vi "Add Caption and Table.vi"(0 "PDF Report IN":T21(xcontrol), 5 "Caption":string, 7 "PdfPTable":refnum<k24>, 11 "error in (no error)":errorcluster) -> (4 "PDF Report OUT":T21(xcontrol), 14 "ms":u32, 15 "error out":errorcluster)   [LabVIEW 2012]
doc: "Version 1.0\nDeveloped by Jean-Marc Simard\nCopyright © 2010, Exaprom Inc.\nAll rights reserved.\nLicense: BSD\n\nWith iTextSharp 4.1.6 (http://itextsharp.sourceforge.net)\nunder Mozilla Public License Version 1.1\n(http://www.mozilla.org/MPL/MPL-1.1.html)"
uses:
  Controls/PDF Report Xcontrol/PDF Report.xctl
  C:/Users/MaxCorp/Documents/TopPerm - Base/DLL/itextsharp.dll
  DLL/itextsharp.dll
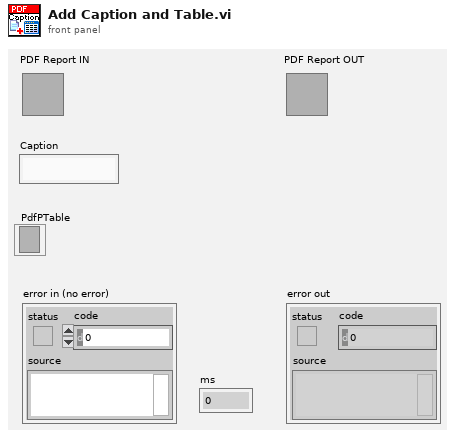
[diagram p1: front panel]
types:
  T1 = typedef "Font cluster.ctl" = cluster{"Name":string, "Size":T2, "Color":T3, "Style":cluster{"Bold":bool, "Italic":bool, "Underline":bool, "Strikeout":bool}}
  T2 = typedef "Font size.ctl" = sgl
  T3 = typedef "Font color.ctl" = u32
  T4 = typedef "Unit.ctl" = enum16{"inch", "mm"}
  T5 = typedef "Paragraphe cluster.ctl" = cluster{" Aligment":T6, "Line spacing":T7}
  T6 = typedef "Texte alignement.ctl" = enum16{"Select", "CENTER", "JUSTIFY", "LEFT", "RIGHT"}
  T7 = typedef "Line spacing.ctl" = enum16{"Select", "1.0", "1.5", "2.0"}
  T8 = typedef "Page dimensions.ctl" = cluster{"Start at page":i32, "Orientation":T9, "widht":sgl, "height":sgl, "Margin left":sgl, "Margin right":sgl, "Margin top":sgl, "Margin bottom":sgl}
  T9 = typedef "Page Orientation.ctl" = enum16{"Portrait", "Landscape"}
  T10 = typedef "Image or Table Caption.ctl" = cluster{"Caption":string, "Separator":string, "Position":enum16{"Above", "Below"}}
  T11 = typedef "Header Footer [ ].ctl" = T12[]
  T12 = typedef "Header Footer cluster.ctl" = cluster{"Start page":i32, "Type":T13, "Alignment":T14, "Vertical Alignement":T15, "Image (%)":sgl, "Page #":T16, "Text":string, "Path":string, "Font":T1, "Font refnum":refnum<k24>, "Line":cluster{"Line":T17, "Thickness (points)":sgl, "Colour":T3}}
  T13 = typedef "Header Footer Type.ctl" = enum16{"Select", "Text", "Text + hyperlink", "Page number", "Image", "Image + hyperlink"}
  T14 = typedef "Header footer horiz alignment.ctl" = enum16{"Left", "Center", "Right"}
  T15 = typedef "Cell Vertical alignment.ctl" = enum16{"TOP", "MIDDLE", "BOTTOM"}
  T16 = typedef "Page number.ctl" = cluster{"Text 1":string, "Text 2":string, "Text 3":string}
  T17 = typedef "Header Footer Line.ctl" = enum16{"No line", "Horizontal line"}
  T18 = typedef "Watermark cluster2.ctl" = cluster{"Show? (F)":bool, "Type":enum16{"Image", "Text"}, "Opacity (%)":sgl, "Rotate(°)":sgl, "Position":cluster{"Position":T19, "X":sgl, "Y":sgl}, "Image path":path, "Scaled(%)":sgl, "Image refnum":refnum<k24>, "Text":string, "Font":cluster{"Name":string, "Size":T2, "Color":T3}, "Font refnum":refnum<k24>, "Alignment":T14, "Automatic":bool}
  T19 = typedef "Watermark Position.ctl" = enum16{"Absolute", "Center (page)", "Center (text section)"}
  T20 = typedef "System Fonts.ctl" = cluster{"Font name [ ]":string[], "Font and file names [ ]":cluster{"Font name":string, "File name":string}[]}
  T21 = cluster{"Document":refnum<k24>, "Writer":refnum<k24>, "Default Font":refnum<k24>, "Default Font cluster":T1, "Path":path, "Unit (default = mm)":T4, "Paragraphe cluster":T5, "Pages dimensions [ ]":T8[], "Captions":cluster{"Image":T10, "Image counter":u16, "Table":T10, "Table counter":u16, "Font":T1}, "Header":T11, "Footer":T11, "Watermark ":T18, "Actual VI name":string, "System Fonts":T20}
  T22 = cluster{"HorizontalAlignment":i32, "SpacingBefore":sgl, "SpacingAfter":sgl}
  T23 = cluster{"HorizontalAlignment":i32, "SpacingAfter":sgl, "SpacingAfter":sgl}
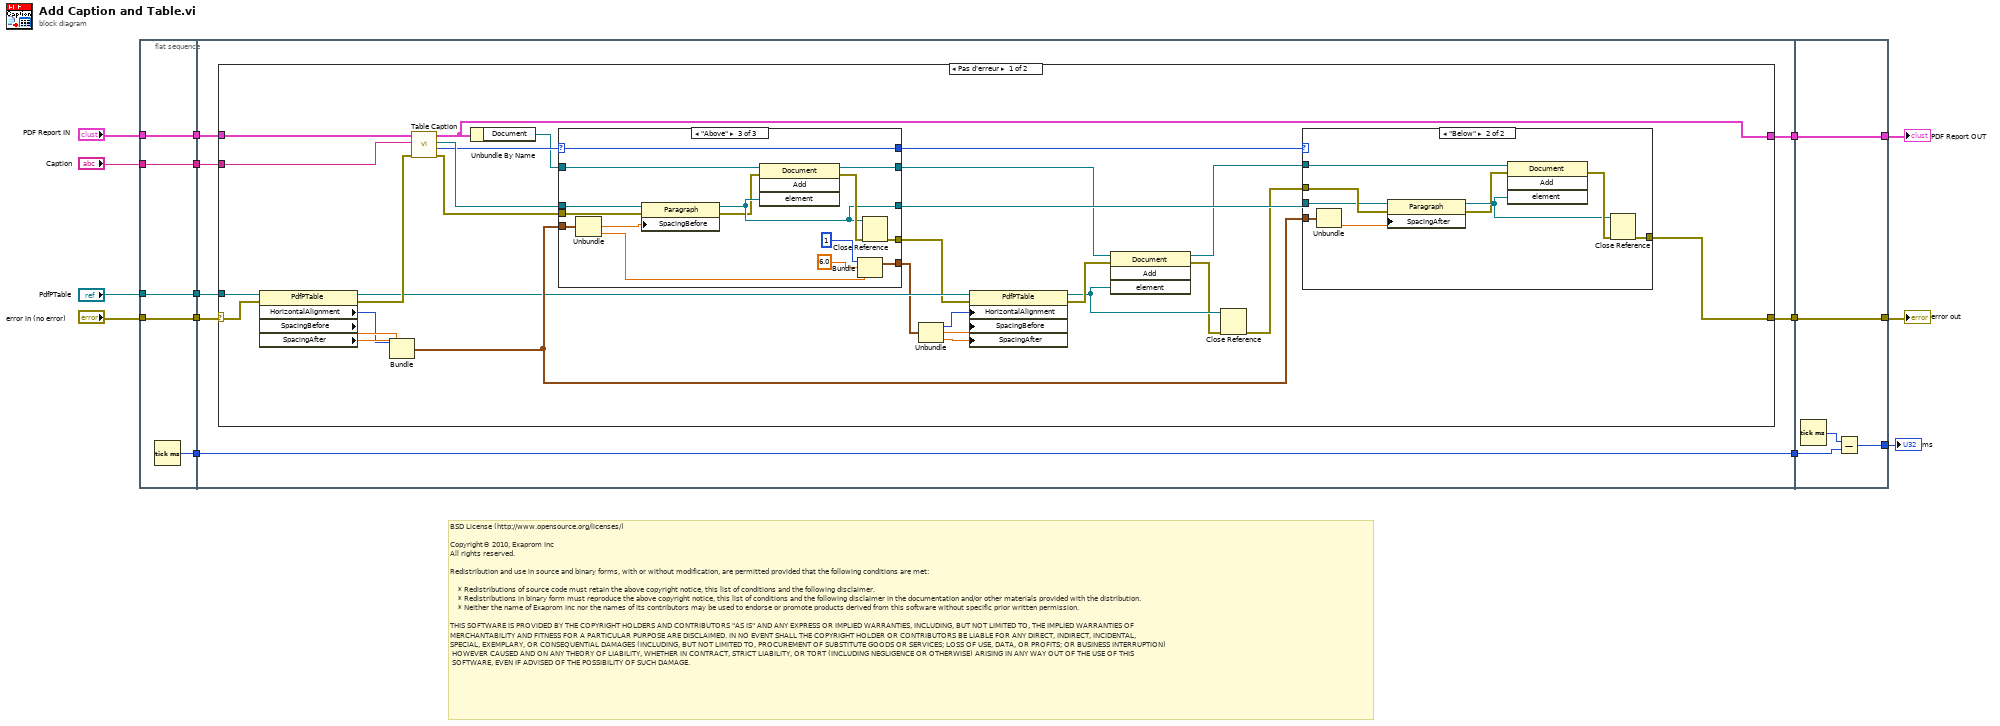
[diagram p0: block diagram]
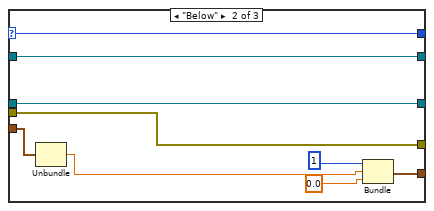
[diagram p4: hidden frame]
diagram:
  # "BSD License (http://www.opensource.org/licenses/)\n\nCopyright© 2010, Exaprom Inc\nAll rights reserved.\n\nRedistribution and use in source and binary forms, with or without modification, are permitted provided that the following conditions are met:\n\n    * Redistributions of source code must retain the above copyright notice, this list of conditions and the following disclaimer.\n    * Redistributions in binary form must reproduce the above copyright notice, this list of conditions and the following disclaimer in the documentation and/or other materials provided with the distribution.\n    * Neither the name of Exaprom Inc nor the names of its contributors may be used to endorse or promote products derived from this software without specific prior written permission.\n\nTHIS SOFTWARE IS PROVIDED BY THE COPYRIGHT HOLDERS AND CONTRIBUTORS \"AS IS\" AND ANY EXPRESS OR IMPLIED WARRANTIES, INCLUDING, BUT NOT LIMITED TO, THE IMPLIED WARRANTIES OF \nMERCHANTABILITY AND FITNESS FOR A PARTICULAR PURPOSE ARE DISCLAIMED. IN NO EVENT SHALL THE COPYRIGHT HOLDER OR CONTRIBUTORS BE LIABLE FOR ANY DIRECT, INDIRECT, INCIDENTAL,\nSPECIAL, EXEMPLARY, OR CONSEQUENTIAL DAMAGES (INCLUDING, BUT NOT LIMITED TO, PROCUREMENT OF SUBSTITUTE GOODS OR SERVICES; LOSS OF USE, DATA, OR PROFITS; OR BUSINESS INTERRUPTION)\n HOWEVER CAUSED AND ON ANY THEORY OF LIABILITY, WHETHER IN CONTRACT, STRICT LIABILITY, OR TORT (INCLUDING NEGLIGENCE OR OTHERWISE) ARISING IN ANY WAY OUT OF THE USE OF THIS\n SOFTWARE, EVEN IF ADVISED OF THE POSSIBILITY OF SUCH DAMAGE."
  n1 = flat-sequence {
    tunnel: "Caption" -> [w17]
    tunnel: "PdfPTable" -> [w18]
    tunnel: "error in (no error)" -> [w19]
    tunnel: "PDF Report IN" -> [w20]
    tunnel: [w20] -> w9
    tunnel: [w19] -> w8
    tunnel: [w18] -> w7
    tunnel: [w17] -> w6
    tunnel: [w16] -> w5
    tunnel: w9 -> [w27]
    tunnel: w8 -> [w24]
    tunnel: w7 -> [w23]
    tunnel: w6 -> [w22]
    tunnel: w5 -> [w21]
    tunnel: [w26] -> w4
    tunnel: [w25] -> w3
    tunnel: [w21] -> w2
    tunnel: [w101] -> w13
    tunnel: [w102] -> w14
    tunnel: w4 -> [w102]
    tunnel: w3 -> [w101]
    tunnel: w2 -> [w100]
    tunnel: [w98] -> w1
    frame #0 {
      n2 = Tick Count (ms)() -> (millisecond timer value=w16:u32)
    }
    frame #1 {
      n3 = case shown="Pas d'erreur" w24 {
        selector: w24 -> [w32 w97]
        tunnel: w27 -> [w31 w96]
        tunnel: [w28 w96] -> w26
        tunnel: [w30 w97] -> w25
        tunnel: w23 -> [w33 _]
        tunnel: w22 -> [w29 _]
        frame No Error {
          n4 = property class="PdfPTable"(reference=w33, error in=w32) -> (reference out=w53:refnum<k24>, error out=w55:errorcluster, "HorizontalAlignment"=w50:i32, "SpacingBefore"=w51:sgl, "SpacingAfter"=w52:sgl)
          n5 = Bundle("HorizontalAlignment"=w50, "SpacingBefore"=w51, "SpacingAfter"=w52) -> (w54:T22)  [unwired: 1 out]
          n6 = call "Table Caption.vi"("error IN"=w55, "Caption IN"=w29, "PDF Report IN"=w31) -> ("error OUT"=w56:errorcluster, "Caption position"=w36:enum16{"No caption", "Above", "Below"}, "Paragraph Refnum"=w37:refnum<k24>, "PDF Report OUT"=w28:T21)  [unwired: 5 out]
          n7 = Unbundle By Name(w28) -> ("Document"=w35:refnum<k24>)
          n8 = case shown="\"Above\"" w36 {
            selector: w36 -> [w68 w77 w91]
            tunnel: w35 -> [w71 w80 w94]
            tunnel: [w71 w80 w93] -> w38
            tunnel: w37 -> [w69 w78 w90]
            tunnel: w56 -> [w70 w79 w87]
            tunnel: [w70 w79 w92] -> w45
            tunnel: [w69 w78 w89] -> w41
            tunnel: [w68 w77 w91] -> w42
            tunnel: w54 -> [w67 w76 w86]
            tunnel: [w67 w75 w84] -> w49
            frame "No caption", Default {
            }
            frame "Below" {
              n9 = Unbundle(w76) -> ("SpacingBefore"=w73:sgl)  [unwired: 2 out]
              n10 = Bundle("HorizontalAlignment"=1, "SpacingBefore"=w73, "SpacingAfter"=sgl 0.0) -> (w75:T22)  [unwired: 1 out]
            }
            frame "Above" {
              n11 = Unbundle(w86) -> ("SpacingBefore"=w85:sgl, "SpacingAfter"=w81:sgl)  [unwired: 1 out]
              n12 = property class="Paragraph"(reference=w90, error in=w87, "SpacingBefore"=w85) -> (reference out=w89:refnum<k24>, error out=w88:errorcluster)
              n13 = invoke class="Document" method="Add"(reference=w94, error in=w88, "element"=w89) -> (reference out=w93:refnum<k24>, error out=w95:errorcluster)  [unwired: 1 in, 2 out]
              n14 = Bundle("HorizontalAlignment"=1, "SpacingAfter"=sgl 6.0, "SpacingAfter"=w81) -> (w84:T23)  [unwired: 1 out]
              n15 = Close Reference(reference=w89, error in (no error)=w95) -> (error out=w92:errorcluster)
            }
          }
          n16 = Unbundle(w49) -> ("HorizontalAlignment"=w46:i32, "SpacingAfter"=w47:sgl, "SpacingAfter"=w48:sgl)
          n17 = property class="PdfPTable"(reference=w53, error in=w45, "HorizontalAlignment"=w46, "SpacingBefore"=w47, "SpacingAfter"=w48) -> (reference out=w43:refnum<k24>, error out=w44:errorcluster)
          n18 = invoke class="Document" method="Add"(reference=w38, error in=w44, "element"=w43) -> (reference out=w39:refnum<k24>, error out=w34:errorcluster)  [unwired: 1 in, 2 out]
          n19 = Close Reference(reference=w43, error in (no error)=w34) -> (error out=w40:errorcluster)
          n20 = case shown="\"Below\"" w42 {
            tunnel: w39 -> [_ w65]
            tunnel: w41 -> [_ w60]
            tunnel: w40 -> [w57 w61]
            tunnel: [w57 w64] -> w30
            tunnel: w54 -> [_ w59]
            frame "No caption", Default {
            }
            frame "Below" {
              n21 = Unbundle(w59) -> ("SpacingAfter"=w58:sgl)  [unwired: 2 out]
              n22 = property class="Paragraph"(reference=w60, error in=w61, "SpacingAfter"=w58) -> (reference out=w63:refnum<k24>, error out=w62:errorcluster)
              n23 = invoke class="Document" method="Add"(reference=w65, error in=w62, "element"=w63) -> (error out=w66:errorcluster)  [unwired: 1 in, 3 out]
              n24 = Close Reference(reference=w63, error in (no error)=w66) -> (error out=w64:errorcluster)
            }
          }
        }
        frame Error {
        }
      }
    }
    frame #2 {
      n25 = Tick Count (ms)() -> (millisecond timer value=w99:u32)
      n26 = Subtract(x=w99, y=w100) -> (x-y=w98:u32)
    }
  }
  "PDF Report OUT" <- w14
  "error out" <- w13
  "ms" <- w1
